vi "LJ_calculate_PWM_parameters.vi"(7 "Duty Cycle (%)":u32=25, 8 "Error In":errorcluster, 9 "Show Confirmation":bool=TRUE, 10 "Laser Rep Rate (Hz)":u32=120, 11 "Laser":enum16{"355nm", "AimingBeam"}(ring)) -> (0 "Error Out":errorcluster, 3 "PWM setting":T1={"DIO_EF_CLOCK1_DIVISOR"=16, "DIO_EF_CLOCK1_ROLL_VALUE"=25000, "DIO#_EF_INDEX"=0, "DIO#_EF_OPTIONS"=1, "DIO#_EF_CONFIG_A"=6250})   [LabVIEW 2020]
uses:
  <vilib>/addons/_JKI.lib/Serialization/JSON/JKI JSON Serialization.lvlib
panel:
  out "Setting path":path
  out "JSON String":string
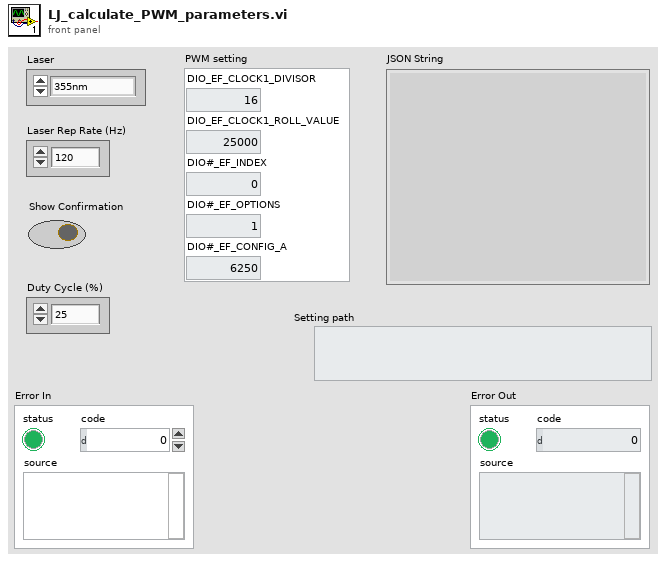
[diagram p1: front panel]
types:
  T1 = cluster{"DIO_EF_CLOCK1_DIVISOR":i16, "DIO_EF_CLOCK1_ROLL_VALUE":i32, "DIO#_EF_INDEX":i16, "DIO#_EF_OPTIONS":i16, "DIO#_EF_CONFIG_A":i32}
  T2 = enum16{"open", "replace", "create", "open or create", "replace or create", "replace or create with confirmation"}
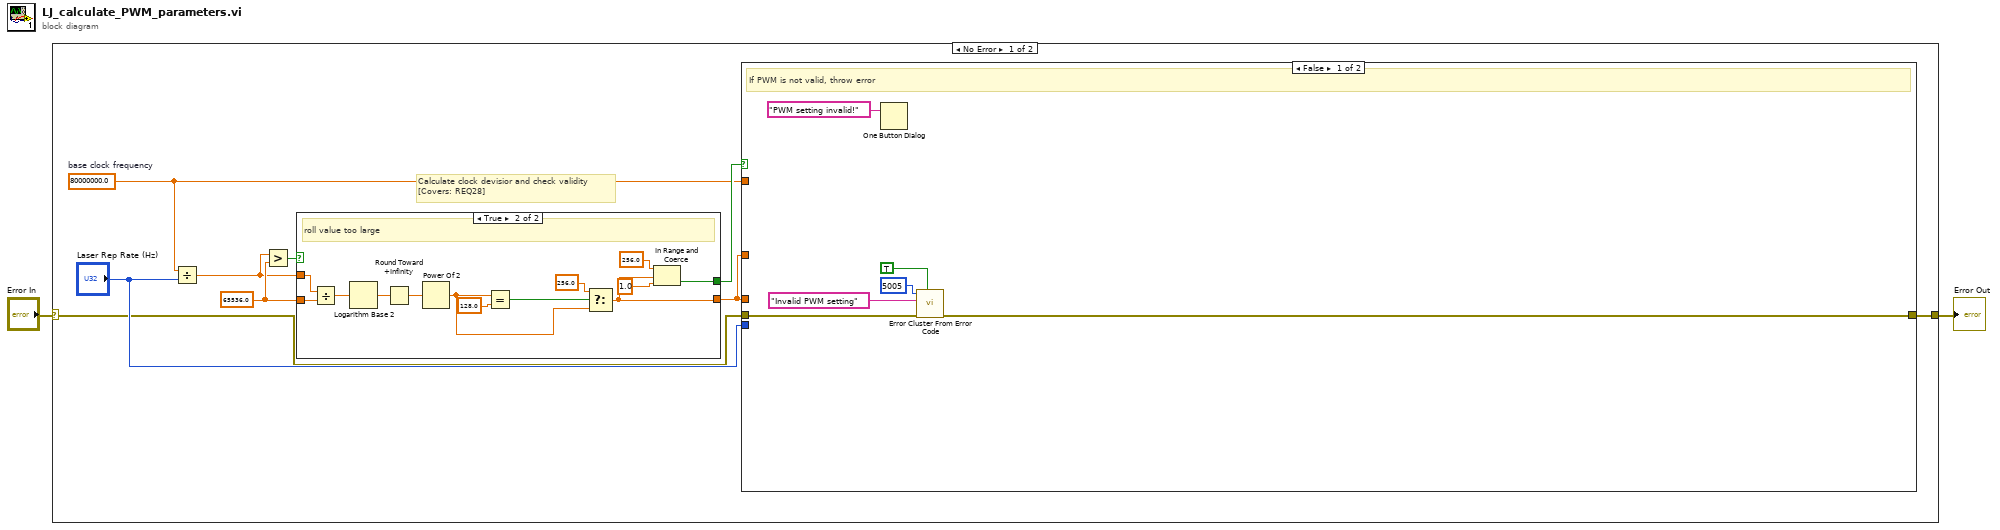
[diagram p0: block diagram]
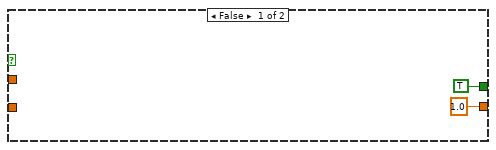
[diagram p2: hidden frame]
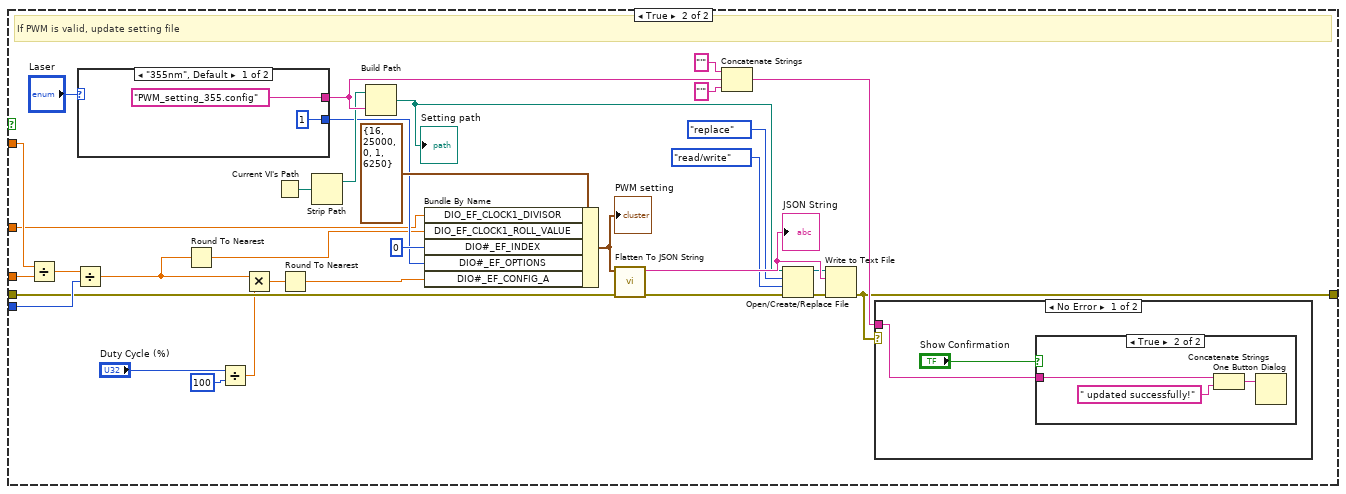
[diagram p3: hidden frame]
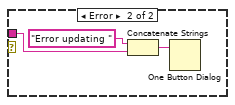
[diagram p5: hidden frame]
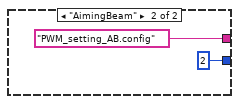
[diagram p6: hidden frame]
diagram:
  n1 = case shown="No Error" "Error In" {
    selector: "Error In" -> [w3 w77]
    tunnel: [w11 w77] -> w1
    frame No Error {
      w9 = 65536.0 ("max roll value")
      w6 = 80000000.0  # base clock frequency
      # "Calculate clock devisior and check validity\n[Covers: REQ28]"
      n2 = Divide(x=w6, y="Laser Rep Rate (Hz)") -> (x/y=w8:dbl)
      n3 = Greater?(x=w8, y=w9) -> (0:w10:bool)
      n4 = case shown="True" w10 {
        tunnel: w9 -> [_ w17]
        tunnel: w8 -> [_ w16]
        tunnel: [TRUE w15] -> w7
        tunnel: [1.0 ("t") w14] -> w5
        frame False {
        }
        frame True {
          # "roll value too large"
          n5 = Divide(x=w16, y=w17) -> (x/y=w22:dbl)
          n6 = Logarithm Base 2(1:w22) -> (0:w23:dbl)
          n7 = Round Toward +Infinity(x=w23) -> (ceil(x): smallest int >= x=w25:dbl)
          n8 = Power Of 2(x=w25) -> (2^x=w26:dbl)
          n9 = Equal?(x=w26, y=128.0) -> (x = y?=w24:bool)
          n10 = Select(t=256.0, s=w24, f=w26) -> (s? t:f=w14:dbl)
          n11 = In Range and Coerce(upper limit=256.0, x=w14, lower limit=1.0) -> (In Range?=w15:bool)  [unwired: 1 out]
        }
      }
      n12 = case shown="False" w7 {
        tunnel: w5 -> [_ w38]
        tunnel: "Laser Rep Rate (Hz)" -> [_ w50]
        tunnel: w5 -> [_ w49]
        tunnel: w6 -> [_ w48]
        tunnel: w3 -> [w27 w47]
        tunnel: [w29 w39] -> w11
        frame False {
          # "If PWM is not valid, throw error"
          n13 = One Button Dialog(message="PWM setting invalid!") -> ()  [unwired: 1 in, 1 out]
          n14 = call <vilib>:"Error Cluster From Error Code.vi"("show call chain? (False)"=TRUE, "error in (no error)"=w27, "error message (\"\")"="Invalid PWM setting" ("error message (\"\")"), "error code (0)"=5005) -> ("error out"=w29:errorcluster)  [unwired: 5 in]
        }
        frame True {
          # "If PWM is valid, update setting file"
          n15 = Divide(x=w48, y=w49) -> (x/y=w55:dbl)
          n16 = Divide(x=w55, y=w50) -> (x/y=w35:dbl)
          n17 = case shown="\"355nm\", Default" "Laser" {
            tunnel: ["PWM_setting_355.config" ("name or relative path") "PWM_setting_AB.config" ("name or relative path")] -> w63
            tunnel: [i16 1 ("DIO#_EF_OPTIONS") i16 2 ("DIO#_EF_OPTIONS")] -> w46
            frame "355nm", Default {
            }
            frame "AimingBeam" {
            }
          }
          n18 = Round To Nearest(number=w35) -> (nearest integer value=w34:dbl)
          n19 = Divide(x="Duty Cycle (%)", y=u32 100) -> (x/y=w33:dbl)
          n20 = Multiply(x=w35, y=w33) -> (x*y=w56:dbl)
          n21 = Current VI's Path() -> (path=w59:path)
          n22 = Round To Nearest(number=w56) -> (nearest integer value=w57:dbl)
          n23 = Strip Path(path=w59) -> (stripped path=w60:path)  [unwired: 1 out]
          n24 = Build Path(base path=w60, name or relative path=w63) -> (appended path=w45:path)
          "Setting path" <- w45
          n25 = Bundle By Name(cluster=T1 {"DIO_EF_CLOCK1_DIVISOR"=16, "DIO_EF_CLOCK1_ROLL_VALUE"=25000, "DIO#_EF_INDEX"=0, "DIO#_EF_OPTIONS"=1, "DIO#_EF_CONFIG_A"=6250} ("PWM setting"), "DIO_EF_CLOCK1_DIVISOR"=w38, "DIO_EF_CLOCK1_ROLL_VALUE"=w34, "DIO#_EF_INDEX"=i16 0, "DIO#_EF_OPTIONS"=w46, "DIO#_EF_CONFIG_A"=w57) -> (w58:T1)
          "PWM setting" <- w58
          n26 = call <vilib>:"Flatten To JSON String.vi"("error in"=w47, "Variant"=w58) -> ("error out"=w41:errorcluster, "JSON String"=w61:string)  [unwired: 8 in]
          "JSON String" <- w61
          n27 = Concatenate Strings("'" ("string"), w63, "'" ("string")) -> (w64:string)
          n28 = Open/Create/Replace File(file path (use dialog)=w45, error in=w41, operation (0:open)=T2."replace", access (0:read/write)=enum16{"read/write", "read-only", "write-only"}."read/write") -> (refnum out=w44:refnum<file>, error out=w40:errorcluster)  [unwired: 2 in, 1 out]
          n29 = Write to Text File(file (use dialog)=w44, text=w61, error in=w40) -> (error out=w39:errorcluster)  [unwired: 1 in, 2 out]
          n30 = case shown="No Error" w39 {
            tunnel: w64 -> [w66 w71]
            frame No Error {
              n31 = case shown="True" "Show Confirmation" {
                tunnel: w66 -> [_ w67]
                frame False {
                }
                frame True {
                  n32 = Concatenate Strings(w67, " updated successfully!" ("string")) -> (w69:string)
                  n33 = One Button Dialog(message=w69) -> ()  [unwired: 1 in, 1 out]
                }
              }
            }
            frame Error {
              n34 = Concatenate Strings("Error updating " ("string"), w71) -> (w70:string)
              n35 = One Button Dialog(message=w70) -> ()  [unwired: 1 in, 1 out]
            }
          }
        }
      }
    }
    frame Error {
    }
  }
  "Error Out" <- w1
